vi "ParentPaletteLinker.vi"   [LabVIEW 2020, in "Defer Panel Updates OpenSource.lvlib"]
uses:
  Defer Panel Updates OpenSource.lvlib
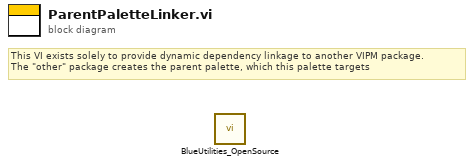
[diagram p0: block diagram]
diagram:
  # "This VI exists solely to provide dynamic dependency linkage to another VIPM package.\nThe \"other\" package creates the parent palette, which this palette targets"
  n1 = call <userlib>:"BlueUtilities_OpenSource.vi"() -> ()  [unwired: 12 in]
